vi "Format InstanceBlockDeviceMappingResponseItemType_LVXML_Loop.vi"(8 "error in (no error)":errorcluster, 10 "Siblings in 3":T2(array[cluster]), 11 "AWS_EC2 in":refnum<class "AWS_EC2.lvclass">) -> (0 "error out":errorcluster, 2 "Array":T3[](array[typedef]), 3 "AWS_EC2 out":refnum<class "AWS_EC2.lvclass">)   [LabVIEW 2014, in "AWS_EC2.lvlib" / "AWS_EC2.lvclass"]
uses:
  AWS_EC2.lvclass
  EC2 Datatypes/InstanceBlockDeviceMappingResponseItemType.ctl
  EC2 Datatypes/EbsInstanceBlockDeviceMappingResponseType.ctl
  lv-xml-parser/r0/trunk/VI Source/EventType.ctl
  AWS_EC2.lvlib
  lv-xml-parser/r0/trunk/VI Source/LV XML Parser.lvlib
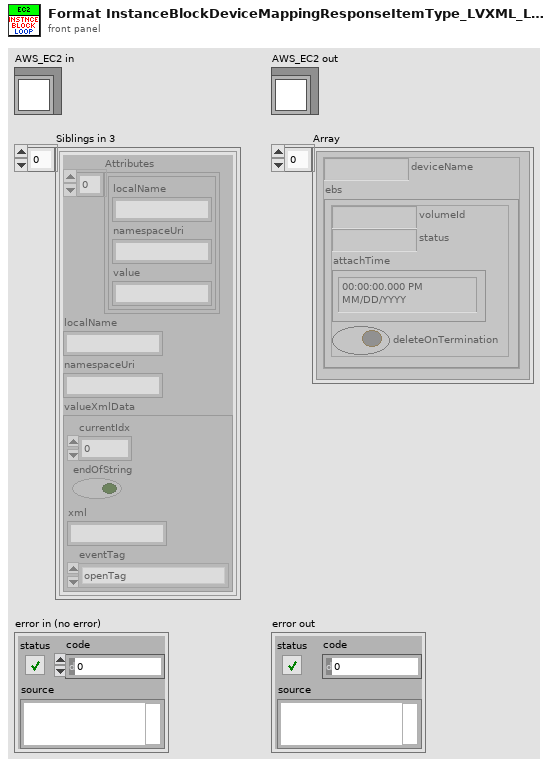
[diagram p1: front panel]
types:
  T1 = typedef "LV XML Parser.lvlib/EventType.ctl" = enum16{"openTag", "endOpenTag", "closeTag", "comment", "endComment", "endOfFile", "attribute", "startXml"}
  T2 = cluster{"Attributes":cluster{"localName":string, "namespaceUri":string, "value":string}[], "localName":string, "namespaceUri":string, "valueXmlData":cluster{"currentIdx":i32, "endOfString":bool, "xml":string, "eventTag":T1}}[]
  T3 = typedef "AWS_EC2.lvlib/InstanceBlockDeviceMappingResponseItemType.ctl" = cluster{"deviceName":string, "ebs":T4}
  T4 = typedef "AWS_EC2.lvlib/EbsInstanceBlockDeviceMappingResponseType.ctl" = cluster{"volumeId":string, "status":string, "attachTime":timestamp, "deleteOnTermination":bool}
  T5 = cluster{"Attributes":cluster{"localName":string, "namespaceUri":string, "value":string}[], "localName":string, "namespaceUri":string, "valueXmlData":cluster{"currentIdx":i32, "endOfString":bool, "xml":string, "eventTag":T1}}
  T6 = cluster{"currentIdx":i32, "endOfString":bool, "xml":string, "eventTag":T1}
  T7 = cluster{"namespaceUri":string, "localName":string}
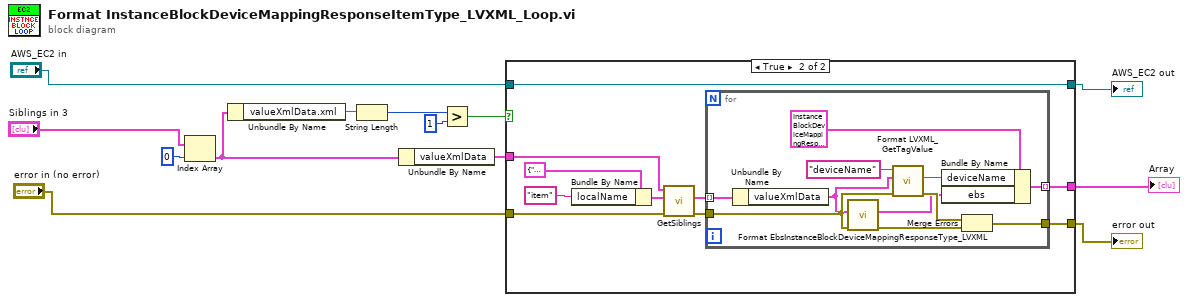
[diagram p0: block diagram]
diagram:
  n1 = Index Array(array="Siblings in 3", index=0) -> (element=w3:T5)
  n2 = Unbundle By Name(w3) -> ("valueXmlData.xml"=w4:string)
  n3 = String Length(string=w4) -> (length=w8:i32)
  n4 = Unbundle By Name(w3) -> ("valueXmlData"=w5:T6)
  n5 = Greater?(x=w8, y=1) -> (0:w6:bool)
  n6 = case shown="True" w6 {
    tunnel: [w15 w24] -> w12
    tunnel: "error in (no error)" -> [w15 w19]
    tunnel: w5 -> [_ w18]
    tunnel: "AWS_EC2 in" -> [w14 w17]
    tunnel: [w14 w17] -> w1
    tunnel: [_ w16] -> w13
    frame False {
    }
    frame True {
      n7 = Bundle By Name(cluster=T7 {"namespaceUri"="", "localName"=""} ("limitToTag"), "localName"="item" ("Tag name")) -> (w21:T7)
      n8 = call "GetSiblings.vi"("error in (no error)"=w19, "limitToTag"=w21, "xmlData"=w18) -> ("error out"=w25:errorcluster, "Siblings"=w22:T2)  [unwired: 7 in]
      n9 = for {
        tunnel: w22 -> [w36] mode=indexing
        tunnel: [w35] -> w24
        tunnel: w25 -> [w28]
        tunnel: [w32] -> w16 mode=indexing
        n10 = Unbundle By Name(w36) -> ("valueXmlData"=w27:T6)
        n11 = call "Format EbsInstanceBlockDeviceMappingResponseType_LVXML.vi"("error in (no error)"=w28, "xmlData in"=w27) -> ("error out"=w29:errorcluster, "EbsInstanceBlockDeviceMappingResponseType"=w26:T4)  [unwired: 7 in, 1 out]
        n12 = call "Format LVXML_GetTagValue.vi"("error in (no error)"=w28, "xmlDataIn"=w27, "Tag name"="deviceName") -> ("error out"=w33:errorcluster, "Value"=w31:string)  [unwired: 6 in, 1 out]
        n13 = Bundle By Name(cluster=T3 {"deviceName"="", "ebs"={"volumeId"="", "status"="", "attachTime"=timestamp(0 s since 1904-01-01), "deleteOnTermination"=FALSE}} ("InstanceBlockDeviceMappingResponseItemType"), "deviceName"=w31, "ebs"=w26) -> (w32:T3)
        n14 = Merge Errors(w33, w29) -> (w35:errorcluster)
      }
    }
  }
  "Array" <- w13
  "error out" <- w12
  "AWS_EC2 out" <- w1
